vi "get_instruction.vi"(11 "client handle":T1) -> (3 "client handle out":T1)   [LabVIEW 2012]
uses:
  <vilib>/httpClient/ClientHandle.ctl
  <vilib>/httpClient/PUTBuffer.vi
  <vilib>/httpClient/LabVIEWHTTPClient.lvlib
panel:
  in  "buffer":string="<?xml version=\"1.0\" encoding=\"utf-8\"?>\n<qm:adaptertask \n  xmlns:qm=\"http://jazz.net/xmlns/alm/qm/v0.1/\"\n  xmlns:alm=\"http://jazz.net/xmlns/alm/v0.1/\"\n  xmlns:dc=\"http://purl.org/dc/elements/1.1/\"\n  xmlns:qmadapter=\"http://jazz.net/xmlns/alm/qm/qmadapter/v0.1\"\n  xmlns:qmresult=\"http://jazz.net/xmlns/alm/qm/v0.1/executionresult/v0.1\"\n  xmlns:qmtask=\"http://jazz.net/xmlns/alm/qm/qmadapter/task/v0.1\"\n  xmlns:atom=\"http://www.w3.org/2005/Atom\"\n  xmlns:xhtml=\"http://www.w3.org/1999/xhtml\"\n  xmlns:rqm=\"http://schema.ibm.com/rqm/2007#executionresult\"\n  xmlns:rqmversion=\"http://jazz.net/xmlns/prod/jazz/rqm/qm/1.0/\"\n>\n<qmtask:progress>100</qmtask:progress>\n<alm:state>com.ibm.rqm.executionframework.common.requeststate.complete</alm:state>\n<qmtask:statusCode>0</qmtask:statusCode>\n</qm:adaptertask>"
  out "body":string
  out "Task type":string
  out "Work available":bool
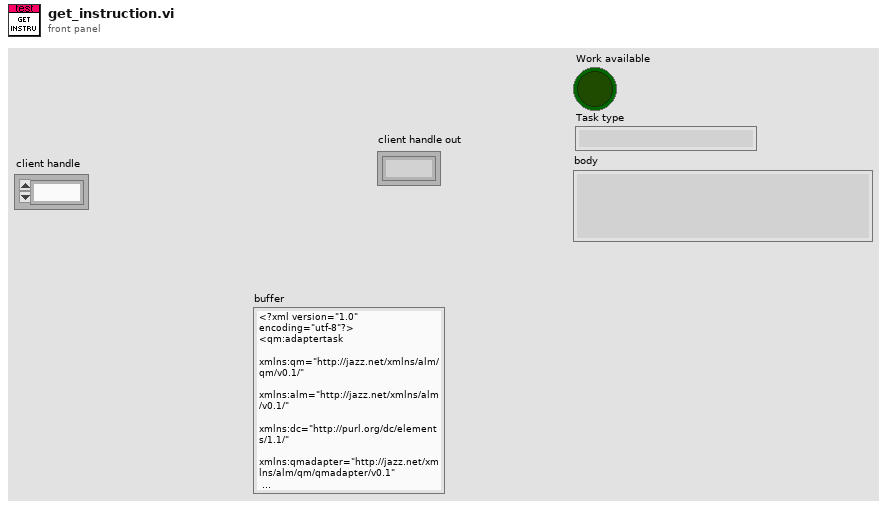
[diagram p1: front panel]
types:
  T1 = typedef "LabVIEWHTTPClient.lvlib/ClientHandle.ctl" = refnum<k1>
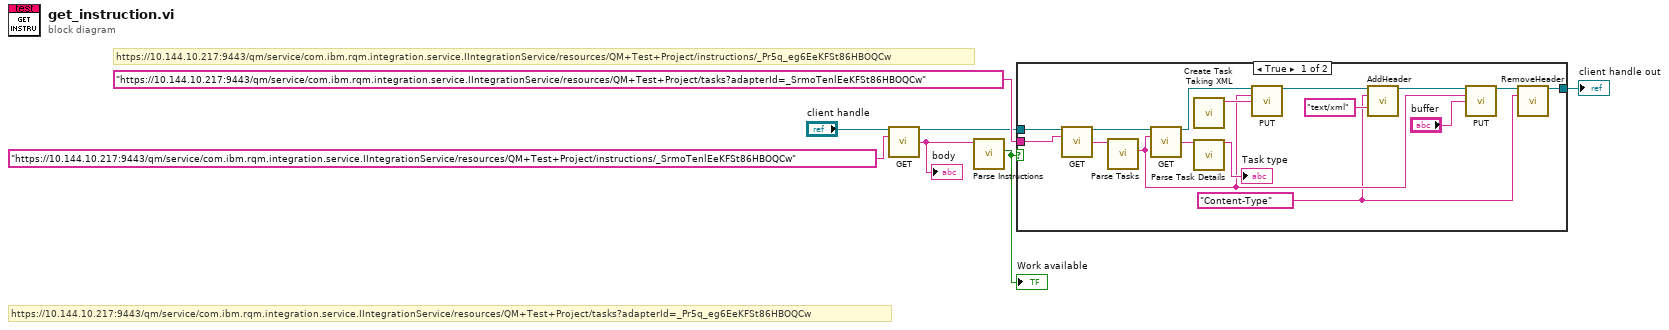
[diagram p0: block diagram]
diagram:
  # "https://10.144.10.217:9443/qm/service/com.ibm.rqm.integration.service.IIntegrationService/resources/QM+Test+Project/tasks?adapterId=_Pr5q_eg6EeKFSt86HBOQCw"
  # "https://10.144.10.217:9443/qm/service/com.ibm.rqm.integration.service.IIntegrationService/resources/QM+Test+Project/instructions/_Pr5q_eg6EeKFSt86HBOQCw"
  n1 = call <vilib>:"GET.vi"("client handle"="client handle", "url"="https://10.144.10.217:9443/qm/service/com.ibm.rqm.integration.service.IIntegrationService/resources/QM+Test+Project/instructions/_SrmoTenlEeKFSt86HBOQCw") -> ("client handle out"=w2:T1, "body"=w5:string)  [unwired: 10 in, 2 out]
  "body" <- w5
  n2 = call "Parse Instructions.vi"("Instructions XML"=w5) -> ("Work available"=w4:bool)  [unwired: 8 in, 2 out]
  "Work available" <- w4
  n3 = case shown="True" w4 {
    tunnel: "https://10.144.10.217:9443/qm/service/com.ibm.rqm.integration.service.IIntegrationService/resources/QM+Test+Project/tasks?adapterId=_SrmoTenlEeKFSt86HBOQCw" ("url") -> [w23 _]
    tunnel: w2 -> [w22 w24]
    tunnel: [w8 w24] -> w1
    frame True {
      w9 = "Content-Type" ("header")
      n4 = call <vilib>:"GET.vi"("client handle"=w22, "url"=w23) -> ("client handle out"=w20:T1, "body"=w21:string)  [unwired: 10 in, 2 out]
      n5 = call "Parse Tasks.vi"("Tasks XML"=w21) -> ("First task URL"=w12:string)  [unwired: 9 in, 1 out]
      n6 = call <vilib>:"GET.vi"("client handle"=w20, "url"=w12) -> ("client handle out"=w16:T1, "body"=w19:string)  [unwired: 10 in, 2 out]
      n7 = call "Create Task Taking XML.vi"() -> ("Take Task XML"=w17:string)  [unwired: 10 in, 1 out]
      n8 = call "Parse Task Details.vi"("Task details XML"=w19) -> ("Task type"=→"Task type":string)  [unwired: 11 in, 7 out]
      n9 = call-poly <vilib>:"PUT.vi"("client handle"=w16, "url"=w12, "buffer"=w17) -> ("client handle out"=w15:T1)  [unwired: 9 in, 3 out]
      n10 = call <vilib>:"AddHeader.vi"("client handle"=w15, "header"=w9, "value"="text/xml") -> ("client handle out"=w13:T1)  [unwired: 11 in, 1 out]
      n11 = call-poly <vilib>:"PUT.vi"("client handle"=w13, "url"=w12, "buffer"="buffer") -> ("client handle out"=w10:T1)  [unwired: 9 in, 3 out]
      n12 = call <vilib>:"RemoveHeader.vi"("client handle"=w10, "header"=w9) -> ("client handle out"=w8:T1)  [unwired: 12 in, 1 out]
    }
    frame False {
    }
  }
  "client handle out" <- w1
